vi "OutBitsTopLevel.vi"   [LabVIEW 2014]
uses:
  OutbitsStateControl.ctl
  <vilib>/rvi/Emulation/niFpgaGetClockAttributes.vi
  <vilib>/rvi/Emulation/niFpgaSctlEmulationGetInTimedLoop.vi
  <vilib>/rvi/Emulation/niFpgaEmulationReportErrorSimple.vi
  <vilib>/rvi/interface/RandomDataEmulation/niFpgaRandomDataHandleErrors.vi
  <vilib>/rvi/Memory/Memory_Emulation/nirvimemoryFastEmulation.vi
  <vilib>/rvi/Memory/Memory_Emulation/nirvimemoryEmulation.vi
  <vilib>/rvi/Emulation/niFpgaEmulationIsFPGAContextNoSignature.vi
  <vilib>/rvi/DataTransferAndStorage/Container/Common/niFpgaContainerGetUniqueNameForEmu.vi
  <vilib>/rvi/Emulation/niFpgaProcessEmulError.vi
  <vilib>/rvi/errors/nirviReportUnexpectedCaseInternalError (U32).vi
  <vilib>/rvi/Emulation/niFpgaCriticalErrorInLSC.vi
  OutbitsGlobalVars.vi
  Sequencer/sequencerGlobVars.vi
  <vilib>/rvi/DataTransferAndStorage/Container/XNode/niFpgaContainer.xnode
  <vilib>/rvi/interface/RandomDataEmulation/nirviRandomDataFpgaReadWriteTemplate.vi
panel:
  # "In rememberence of the most famous Outbits in COLLAPS MCP program\nthis is the toplevel module to also have them in TILDA.\n\nThere will be three Outbits. each can be set either to:\n - toggle (track, scan or step)\n - on/off (track, scan or step)\n\nThe Outbits will be put out on DIOs:\n - Connector1/DIO3 \n - Connector1/DIO4 \n - Connector1/DIO5\n\nMore Details see OneNote documentary"
types:
  T1 = typedef "OutbitsStateControl.ctl" = enum16{"Init", "Idle", "loading", "listening", "clearing", "error"}
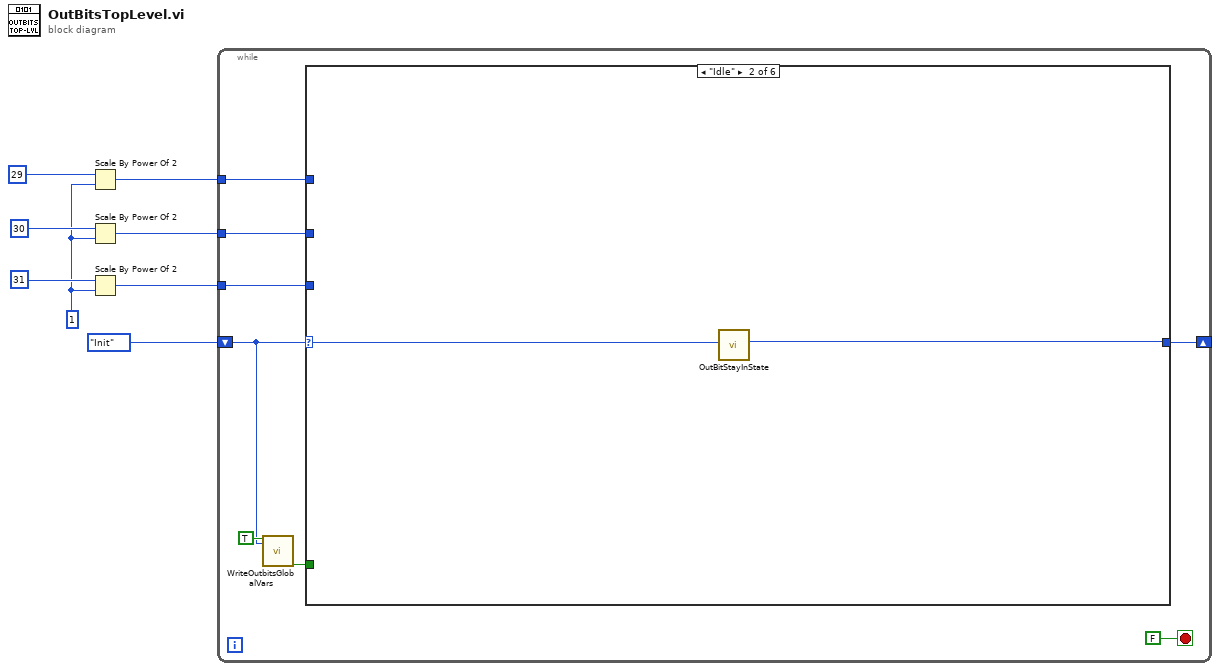
[diagram p0: block diagram]
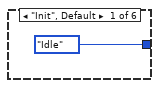
[diagram p2: hidden frame]
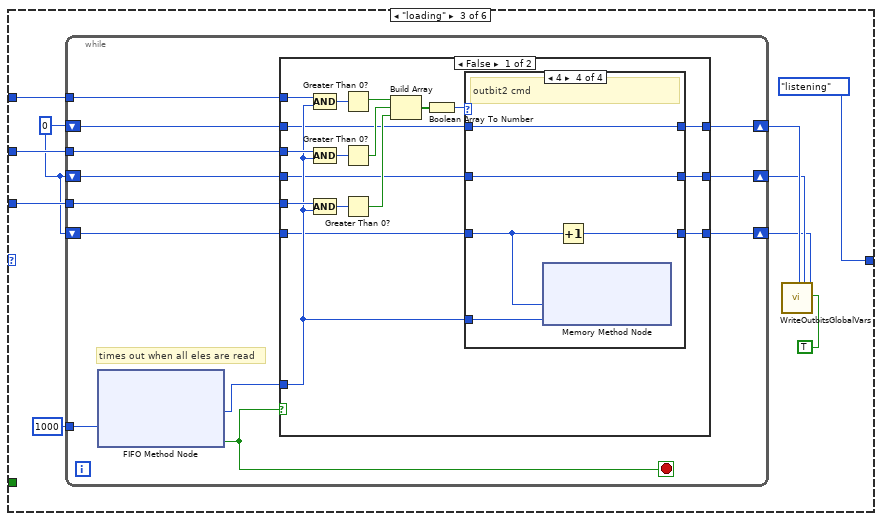
[diagram p3: hidden frame]
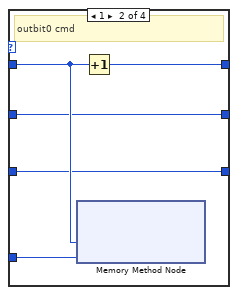
[diagram p5: hidden frame]
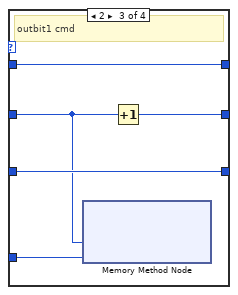
[diagram p6: hidden frame]
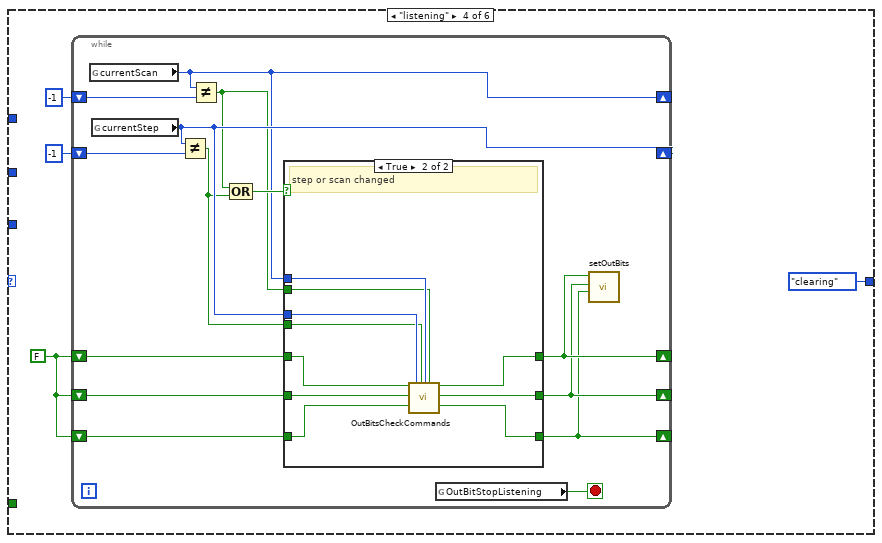
[diagram p8: hidden frame]
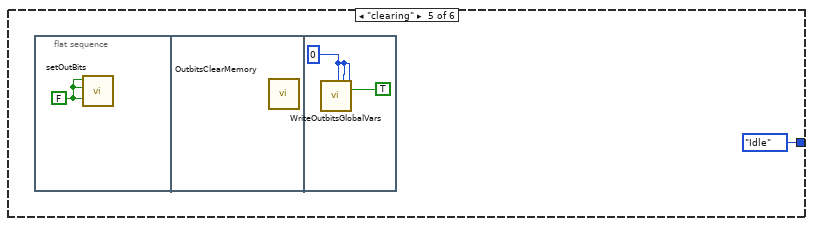
[diagram p10: hidden frame]
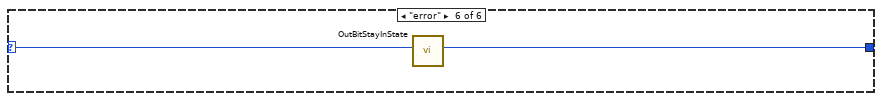
[diagram p11: hidden frame]
diagram:
  w2 = u32 1 ("Element")
  n1 = Scale By Power Of 2(n=i16 29, x=w2) -> (x*2^n=w4:u32)
  n2 = Scale By Power Of 2(n=i16 30, x=w2) -> (x*2^n=w3:u32)
  n3 = Scale By Power Of 2(n=i16 31, x=w2) -> (x*2^n=w1:u32)
  n4 = while {
    shift-right: [w13] -> _
    shift-left: OutbitsStateControl."Init" ("OutBitsState") -> [w14]
    tunnel: w4 -> [w12]
    tunnel: w3 -> [w11]
    tunnel: w1 -> [w10]
    stop <- FALSE stop-if-true
    n5 = call "WriteOutbitsGlobalVars.vi"("writeState"=TRUE, "OutBitsState"=w14) -> ("done"=w9:bool)  [unwired: 17 in]
    n6 = case shown="\"Idle\"" w14 {
      selector: w14 -> [_ w19 _ _ _ w117]
      tunnel: [OutbitsStateControl."Idle" ("OutBitsState") w18 OutbitsStateControl."listening" ("OutBitsStateNext") OutbitsStateControl."clearing" ("OutBitsStateNext") OutbitsStateControl."Idle" ("OutBitsStateNext") w116] -> w13
      tunnel: w12 -> [_ _ w28 _ _ _]
      tunnel: w11 -> [_ _ w27 _ _ _]
      tunnel: w10 -> [_ _ w26 _ _ _]
      tunnel: w9 -> [_ _ _ _ _ _]
      frame "Init", Default {
      }
      frame "Idle" {
        n7 = call "OutBitStayInState.vi"("OutBitsStateBefore"=w19) -> ("OutBitsStateNext"=w18:T1)  [unwired: 10 in]
      }
      frame "loading" {
        w25 = u32 0 ("Address")
        n8 = while {
          tunnel: 1000 ("Timeout") -> [w41]
          tunnel: w28 -> [w38]
          tunnel: w27 -> [w37]
          tunnel: w26 -> [w36]
          shift-right: [w34] -> w24
          shift-left: w25 -> [w35]
          shift-right: [w33] -> w23
          shift-left: w25 -> [w32]
          shift-right: [w31] -> w22
          shift-left: w25 -> [w30]
          stop <- w40 stop-if-true
          # "times out when all eles are read"
          n9 = xnode ("FIFO Method Node")("Timeout"=w41) -> ("Element"=w39:u32, "Timed Out?"=w40:bool)  [unwired: 1 in, 1 out]
          n10 = case shown="False" w40 {
            tunnel: w39 -> [w48 _]
            tunnel: w38 -> [w59 _]
            tunnel: w37 -> [w56 _]
            tunnel: w36 -> [w54 _]
            tunnel: w35 -> [w47 w80]
            tunnel: [w46 w80] -> w34
            tunnel: [w45 w79] -> w33
            tunnel: w32 -> [w44 w79]
            tunnel: [w43 w78] -> w31
            tunnel: w30 -> [w42 w78]
            frame False {
              n11 = Compound Arithmetic op=AND(w59, w48) -> (w58:u32)
              n12 = Compound Arithmetic op=AND(w56, w48) -> (w57:u32)
              n13 = Compound Arithmetic op=AND(w54, w48) -> (w55:u32)
              n14 = Greater Than 0?(x=w58) -> (x > 0?=w53:bool)
              n15 = Greater Than 0?(x=w57) -> (x > 0?=w52:bool)
              n16 = Greater Than 0?(x=w55) -> (x > 0?=w51:bool)
              n17 = Build Array(w53, w52, w51) -> (w50:bool[])
              n18 = Boolean Array To Number(Boolean array=w50) -> (number=w49:u8)
              n19 = case shown="4" w49 {
                tunnel: w48 -> [_ w67 w71 w76]
                tunnel: w47 -> [w62 w66 w69 w77]
                tunnel: [w62 w65 w69 w77] -> w46
                tunnel: [w61 w64 w68 w74] -> w45
                tunnel: w44 -> [w61 w64 w70 w74]
                tunnel: [w60 w63 w72 w73] -> w43
                tunnel: w42 -> [w60 w63 w72 w75]
                frame 0, Default {
                }
                frame 1 {
                  # "outbit0 cmd"
                  n20 = xnode ("Memory Method Node")("Address"=w66, "Data"=w67) -> ()  [unwired: 1 in, 1 out]
                  n21 = Increment(x=w66) -> (x+1=w65:u32)
                }
                frame 2 {
                  # "outbit1 cmd"
                  n22 = xnode ("Memory Method Node")("Address"=w70, "Data"=w71) -> ()  [unwired: 1 in, 1 out]
                  n23 = Increment(x=w70) -> (x+1=w68:u32)
                }
                frame 4 {
                  # "outbit2 cmd"
                  n24 = xnode ("Memory Method Node")("Address"=w75, "Data"=w76) -> ()  [unwired: 1 in, 1 out]
                  n25 = Increment(x=w75) -> (x+1=w73:u32)
                }
              }
            }
            frame True {
              # "timed out"
            }
          }
        }
        n26 = call "WriteOutbitsGlobalVars.vi"("nOfCmdsOutbit0"=w24, "nOfCmdsOutbit1"=w23, "nOfCmdsOutbit2"=w22, "write_nOfCmdsOutbitsAll"=TRUE) -> ()  [unwired: 15 in, 1 out]
      }
      frame "listening" {
        w82 = FALSE
        n27 = while {
          shift-right: [w93] -> _
          shift-left: -1 ("currentScan") -> [w97]
          shift-right: [w94] -> _
          shift-left: -1 ("currentStep") -> [w96]
          shift-right: [w87] -> _
          shift-left: w82 -> [w90]
          shift-right: [w86] -> _
          shift-left: w82 -> [w89]
          shift-right: [w85] -> _
          shift-left: w82 -> [w88]
          stop <- w98 stop-if-true
          n28 = global read "sequencerGlobVars.vi" "currentScan"() -> (w93:i32)
          n29 = global read "sequencerGlobVars.vi" "currentStep"() -> (w94:i32)
          n30 = Not Equal?(x=w94, y=w96) -> (x != y?=w92:bool)
          n31 = Not Equal?(x=w93, y=w97) -> (x != y?=w91:bool)
          n32 = Compound Arithmetic op=OR(w91, w92) -> (w95:bool)
          n33 = case shown="True" w95 {
            tunnel: w94 -> [_ w105]
            tunnel: w93 -> [_ w103]
            tunnel: w92 -> [_ w104]
            tunnel: w91 -> [_ w102]
            tunnel: w90 -> [w101 w109]
            tunnel: w89 -> [w100 w111]
            tunnel: w88 -> [w99 w110]
            tunnel: [w101 w108] -> w87
            tunnel: [w100 w107] -> w86
            tunnel: [w99 w106] -> w85
            frame False {
            }
            frame True {
              # "step or scan changed"
              n34 = call "OutBitsCheckCommands.vi"("outBit0"=w109, "outBit1"=w111, "outBit2"=w110, "actStep"=w105, "stepChanged"=w104, "actScan"=w103, "scanChanged"=w102) -> ("outBit0out"=w108:bool, "outBit1out"=w107:bool, "outBit2out"=w106:bool)  [unwired: 10 in]
            }
          }
          n35 = global read "OutbitsGlobalVars.vi" "OutBitStopListening"() -> (w98:bool)
          n36 = call "setOutBits.vi"("outBit2"=w85, "outBit1"=w86, "outBit0"=w87) -> ()  [unwired: 9 in]
        }
      }
      frame "clearing" {
        n37 = flat-sequence {
          frame #0 {
            w113 = FALSE ("outBit0")
            n38 = call "setOutBits.vi"("outBit2"=w113, "outBit1"=w113, "outBit0"=w113) -> ()  [unwired: 9 in]
          }
          frame #1 {
            n39 = call "OutbitsClearMemory.vi"() -> ()  [unwired: 12 in]
          }
          frame #2 {
            w114 = u32 0 ("nOfCmdsOutbit0")
            n40 = call "WriteOutbitsGlobalVars.vi"("nOfCmdsOutbit0"=w114, "nOfCmdsOutbit1"=w114, "nOfCmdsOutbit2"=w114, "write_nOfCmdsOutbitsAll"=TRUE) -> ()  [unwired: 15 in, 1 out]
          }
        }
      }
      frame "error" {
        n41 = call "OutBitStayInState.vi"("OutBitsStateBefore"=w117) -> ("OutBitsStateNext"=w116:T1)  [unwired: 10 in]
      }
    }
  }
